vi "MB Serial Master Query.vi"(4 "Timeout":u32=10000, 6 "Serial Parameters":T1 {"Slave Address" format="%.0x"}, 7 "Modbus Data Unit In":T3={"function"=1, "Data"=[]} {"function" items=["Read Discrete Inputs"=2, "Read Coils"=1, "Write Single Coil"=5, "Write Multiple Coils"=15, "Read Input Register"=4, "Read Holding Registers"=3, "Write Single Register"=6, "Write Multiple Registers"=16, "Read/Write Multiple Registers"=23, "Mask Write Register"=22, "Read FIFO Queue"=24, "Read File Record"=20, "Write File Record"=21, "Read Exception Status"=7, "Diagnostic"=8, "Get Com Event Counter"=11, "Get Com Event Log"=12, "Report Slave ID"=17, "Read Device Identification"=43]; "Data" format="%.0x"}, 8 "error in (no error)":errorcluster, 9 "Use MODBUS Data Unit?":bool, 10 "Modbus Command":T2={"Function Code"=1, "Starting Address"=0, "Quantity"=0, "Data"=[], "Discrete"=[]} {"Function Code" items=["Read Coils"=1, "Read Discrete Inputs"=2, "Read Holding Registers"=3, "Read Input Registers"=4, "Write Single Coil"=5, "Write Single Register"=6, "Read Exception Status"=7, "Write Multiple Coils"=15, "Write Multiple Registers"=16]}, 11 "VISA resource name":refnum<visa-resource-name>) -> (0 "error out":errorcluster, 1 "Exception Code":u8 format="%.0x", 2 "Registers":cluster{"Registers":u16[], "Discrete":bool[]}, 3 "VISA resource name out":refnum<visa-resource-name>, 5 "Modbus Data Unit Out":T3={"function"=1, "Data"=[]} {"function" items=["Read Discrete Inputs"=2, "Read Coils"=1, "Write Single Coil"=5, "Write Multiple Coils"=15, "Read Input Register"=4, "Read Holding Registers"=3, "Write Single Register"=6, "Write Multiple Registers"=16, "Read/Write Multiple Registers"=23, "Mask Write Register"=22, "Read FIFO Queue"=24, "Read File Record"=20, "Write File Record"=21, "Read Exception Status"=7, "Diagnostic"=8, "Get Com Event Counter"=11, "Get Com Event Log"=12, "Report Slave ID"=17, "Read Device Identification"=43]; "Data" format="%.0x"})   [LabVIEW 2019, in "NI_modbus_upd.lvlib"]
uses:
  NI_modbus_upd.lvlib
  Ctl/MB Modbus Data Unit.ctl
  Modbus Data Unit (PDU)/Function.ctl
  Ctl/MB Modbus Command.ctl
panel:
  # "VI Name: MB Serial Master Query.vi\nPurpose: Performs a Modbus query."
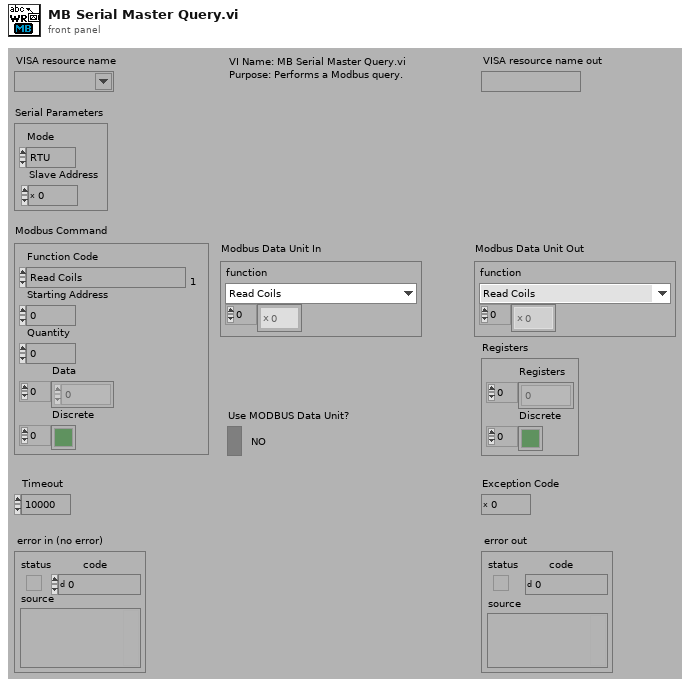
[diagram p1: front panel]
types:
  T1 = cluster{"Mode":enum16{"RTU", "ASCII"}, "Slave Address":u8}
  T2 = typedef "NI_modbus_upd.lvlib/MB Modbus Command.ctl" = cluster{"Function Code":u8, "Starting Address":u16, "Quantity":u16, "Data":u16[], "Discrete":bool[]}
  T3 = typedef "NI_modbus_upd.lvlib/MB Modbus Data Unit.ctl" = cluster{"function":T4, "Data":u8[]}
  T4 = typedef "NI_modbus_upd.lvlib/Function.ctl" = u8
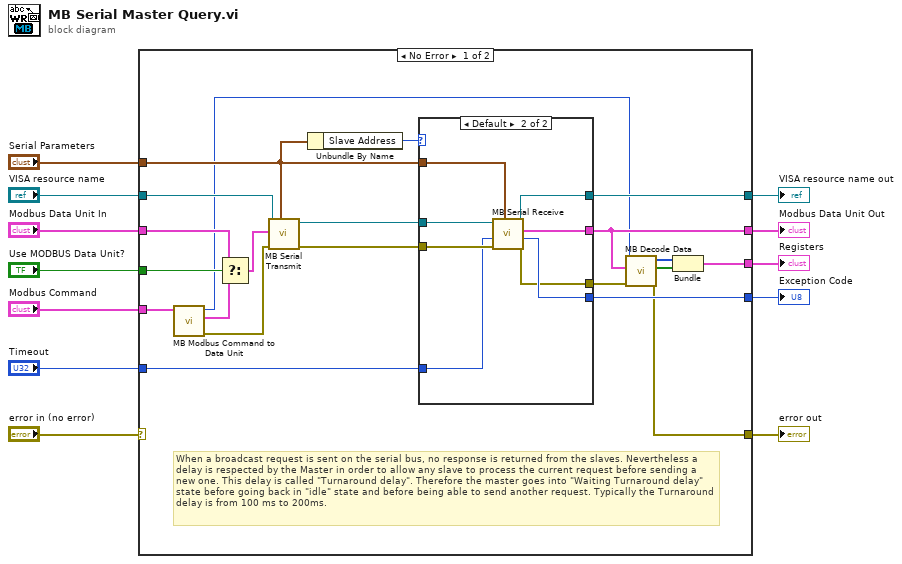
[diagram p0: block diagram]
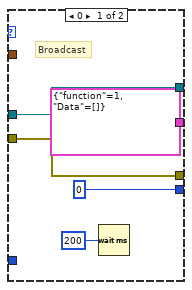
[diagram p2: hidden frame]
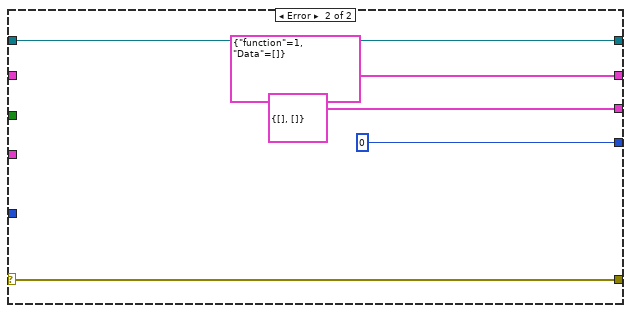
[diagram p3: hidden frame]
diagram:
  n1 = case shown="No Error" "error in (no error)" {
    selector: "error in (no error)" -> [_ w47]
    tunnel: [w26 T3 {"function"=1, "Data"=[]} ("MODBUS Data Unit")] -> w5
    tunnel: [w30 u8 0 ("Exception Code")] -> w12
    tunnel: [w24 w47] -> w3
    tunnel: "VISA resource name" -> [w33 w51]
    tunnel: "Timeout" -> [w32 _]
    tunnel: [w31 w51] -> w9
    tunnel: "Modbus Data Unit In" -> [w29 _]
    tunnel: "Use MODBUS Data Unit?" -> [w28 _]
    tunnel: "Modbus Command" -> [w27 _]
    tunnel: [w25 cluster{"Registers":u16[], "Discrete":bool[]} {"Registers"=[], "Discrete"=[]}] -> w4
    tunnel: "Serial Parameters" -> [w16 _]
    frame No Error {
      # "When a broadcast request is sent on the serial bus, no response is returned from the slaves. Nevertheless a delay is respected by the Master in order to allow any slave to process the current request before sending a new one. This delay is called \"Turnaround delay\". Therefore the master goes into \"Waiting Turnaround delay\" state before going back in \"idle\" state and before being able to send another request. Typically the Turnaround delay is from 100 ms to 200ms."
      n2 = call "MB Modbus Command to Data Unit.vi"("Modbus Command"=w27) -> ("error out"=w13:errorcluster, "Modbus Data Unit"=w15:T3, "Quantity"=w14:u16)  [unwired: 8 in]
      n3 = Select(t=w29, s=w28, f=w15) -> (s? t:f=w17:T3)
      n4 = call "MB Serial Transmit.vi"("Serial Parameters"=w16, "error in (no error)"=w13, "Modbus Data Unit"=w17, "VISA resource name"=w33) -> ("error out"=w22:errorcluster, "VISA resource name out"=w23:refnum<visa-resource-name>)  [unwired: 6 in]
      n5 = Unbundle By Name(w16) -> ("Slave Address"=w21:u8)
      n6 = case shown="Default" w21 {
        tunnel: w23 -> [w38 w46]
        tunnel: w22 -> [w35 w45]
        tunnel: w32 -> [_ w44]
        tunnel: w16 -> [_ w43]
        tunnel: [w38 w42] -> w31
        tunnel: [u8 0 ("Exception Code") w41] -> w30
        tunnel: [T3 {"function"=1, "Data"=[]} ("MODBUS Data Unit") w40] -> w26
        tunnel: [w35 w39] -> w20
        frame 0 {
          # "Broadcast"
          n7 = Wait (ms)(milliseconds to wait=u32 200) -> ()  [unwired: 1 out]
        }
        frame Default {
          n8 = call "MB Serial Receive.vi"("Serial Parameters"=w43, "error in (no error)"=w45, "Timeout"=w44, "VISA resource name"=w46) -> ("error out"=w39:errorcluster, "Exception Code"=w41:u8, "Modbus Data Unit"=w40:T3, "VISA resource name out"=w42:refnum<visa-resource-name>)  [unwired: 4 in]
        }
      }
      n9 = call "MB Decode Data.vi"("error in (no error)"=w20, "Response MDU"=w26, "Function Code"=w14) -> ("error out"=w24:errorcluster, "Discrete"=w18:bool[], "Registers"=w19:u16[])  [unwired: 6 in]
      n10 = Bundle("Registers"=w19, "Discrete"=w18) -> (w25:cluster{"Registers":u16[], "Discrete":bool[]})  [unwired: 1 in]
    }
    frame Error {
    }
  }
  "error out" <- w3
  "Exception Code" <- w12
  "VISA resource name out" <- w9
  "Modbus Data Unit Out" <- w5
  "Registers" <- w4
